vi "password.vi"   [LabVIEW 2012]
uses:
  <vilib>/addons/internet/NI_InternetTK_Common_VIs.lvlib
  <vilib>/addons/internet/NI_InternetTK_Core_VIs.lvlib
types:
  T1 = typedef "CGI Connection Info.ctl" = cluster{"name":string, "type":T2, "session":T3}
  T2 = typedef "CGI Request Type.ctl" = enum16{"cgi", ".spool first", ".spool", ".spool last"}
  T3 = typedef "HTTP Session.ctl" = refnum<k1>
  T4 = typedef "NI_FTP.lvlib/Keyed Array.ctl" = cluster{"keys":string[], "values":string[]}
  T5 = enum16{"(default)", "monospaced", "italic", "bold", "underlined", "strike-through", "big", "small", "superscript", "subscript"}
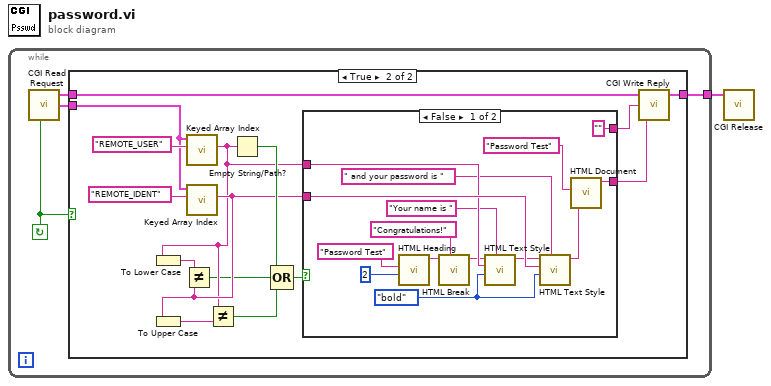
[diagram p0: block diagram]
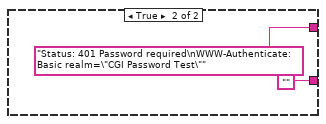
[diagram p3: hidden frame]
diagram:
  n1 = while {
    tunnel: [w4] -> w1
    stop <- w2 continue-if-true
    n2 = call <vilib>:"CGI Read Request.vi"() -> ("valid request?"=w2:bool, "cgi connection info"=w5:T1, "env"=w3:T4)  [unwired: 4 in, 1 out]
    n3 = case shown="True" w2 {
      tunnel: w5 -> [w6 w21]
      tunnel: [w6 w20] -> w4
      tunnel: w3 -> [_ w13]
      frame False {
      }
      frame True {
        n4 = call <vilib>:"Keyed Array Index.vi"("key"="REMOTE_USER" ("name"), "array in"=w13) -> ("value"=w9:string)  [unwired: 3 in, 2 out]
        n5 = To Lower Case(string=w9) -> (all lower case string=w12:string)
        n6 = call <vilib>:"Keyed Array Index.vi"("key"="REMOTE_IDENT" ("name"), "array in"=w13) -> ("value"=w11:string)  [unwired: 3 in, 2 out]
        n7 = To Upper Case(1:w11) -> (0:w10:string)
        n8 = Not Equal?(x=w12, y=w11) -> (x != y?=w8:bool)
        n9 = Not Equal?(x=w9, y=w10) -> (x != y?=w7:bool)
        n10 = Empty String/Path?(string/path=w9) -> (empty?=w14:bool)
        n11 = Compound Arithmetic op=OR(w14, w8, w7) -> (w15:bool)
        n12 = case shown="False" w15 {
          tunnel: w9 -> [w31 _]
          tunnel: w11 -> [w33 _]
          tunnel: ["" "Status: 401 Password required\nWWW-Authenticate: Basic realm=\"CGI Password Test\""] -> w18
          tunnel: [w34 ""] -> w19
          frame False {
            w32 = T5."bold" ("style")
            n13 = call <vilib>:"HTML Heading.vi"("level (1)"=2, "heading"="Password Test") -> ("HTML out"=w24:string)  [unwired: 9 in]
            n14 = call <vilib>:"HTML Break.vi"("label"="Congratulations!" ("heading"), "HTML in"=w24) -> ("HTML out"=w23:string)  [unwired: 9 in]
            n15 = call <vilib>:"HTML Text Style.vi"("label"="Your name is " ("heading"), "style (default)"=w32, "text"=w31, "HTML in"=w23) -> ("HTML out"=w26:string)  [unwired: 7 in]
            n16 = call <vilib>:"HTML Text Style.vi"("label"=" and your password is " ("heading"), "style (default)"=w32, "text"=w33, "HTML in"=w26) -> ("HTML out"=w25:string)  [unwired: 7 in]
            n17 = call <vilib>:"HTML Document.vi"("document body"=w25, "document title"="Password Test") -> ("HTML Document"=w34:string)  [unwired: 9 in]
          }
          frame True {
          }
        }
        n18 = call <vilib>:"CGI Write Reply.vi"("content"=w19, "header"=w18, "cgi connection info"=w21) -> ("cgi connection info out"=w20:T1)  [unwired: 2 in]
      }
    }
  }
  n19 = call <vilib>:"CGI Release.vi"("cgi connection info"=w1) -> ()  [unwired: 5 in]
